vi "Create HTML.vi"(7 "FP Reference":refnum<class "Web Front Panel.lvclass">, 8 "error in (no error)":errorcluster, 10 "VI Identifier":string, 11 "Text In":refnum<class "Text.lvclass">) -> (0 "error out":errorcluster, 1 "js code for controls":string, 2 "js variables":string, 3 "Text Out":refnum<class "Text.lvclass">, 4 "script dependencies":string[](array[string]), 5 "HTML":string, 6 "js code for indicators":string)   [LabVIEW 2017, in "Front Panel Publisher.lvlib" / "Text.lvclass"]
uses:
  Text.lvclass
  Object_class/Object.lvclass
  Front Panel Publisher.lvlib
  String_class/String.lvclass
  Web Front Panel_class/Web Front Panel.lvclass
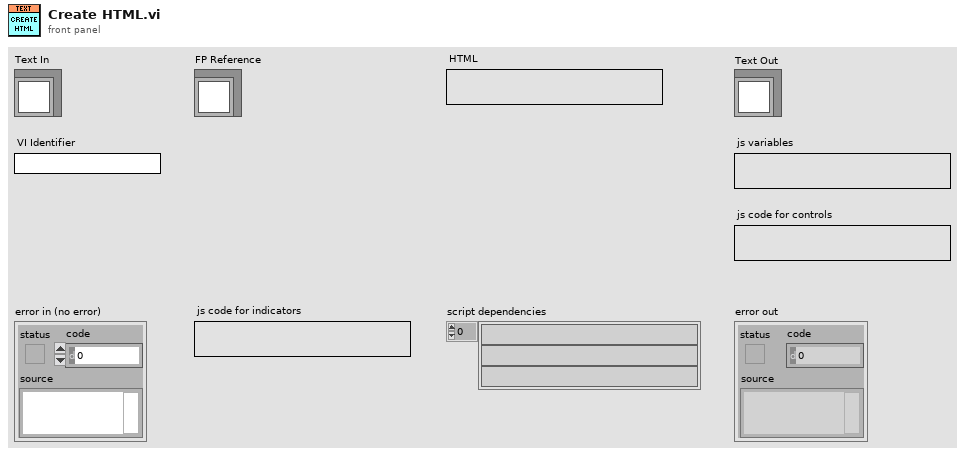
[diagram p1: front panel]
types:
  T1 = typedef "Front Panel Publisher.lvlib/Object.lvclass/Attributes.ctl" = cluster{"UID":i32, "Type":string, "Starting Location":T2, "Reference":refnum<vi>, "Cluster Component":bool, "Starting Rect Position":cluster{"Left":i16, "Top":i16}, "Owning Pane":refnum<vi>, "Master Total Rect Delta":T3}
  T2 = typedef "Front Panel Publisher.lvlib/Object.lvclass/Coordinates.ctl" = cluster{"Left":i32, "Top":i32, "Height":u32, "Width":u32}
  T3 = typedef "LVRectTypeDef.ctl" = cluster{"Left":i16, "Top":i16, "Right":i16, "Bottom":i16}
  T4 = typedef "Front Panel Publisher.lvlib/Text.lvclass/Attributes.ctl" = cluster{"Text":string, "Font":string, "Font Size":u32, "Visible":bool, "Control Reference":refnum<vi>}
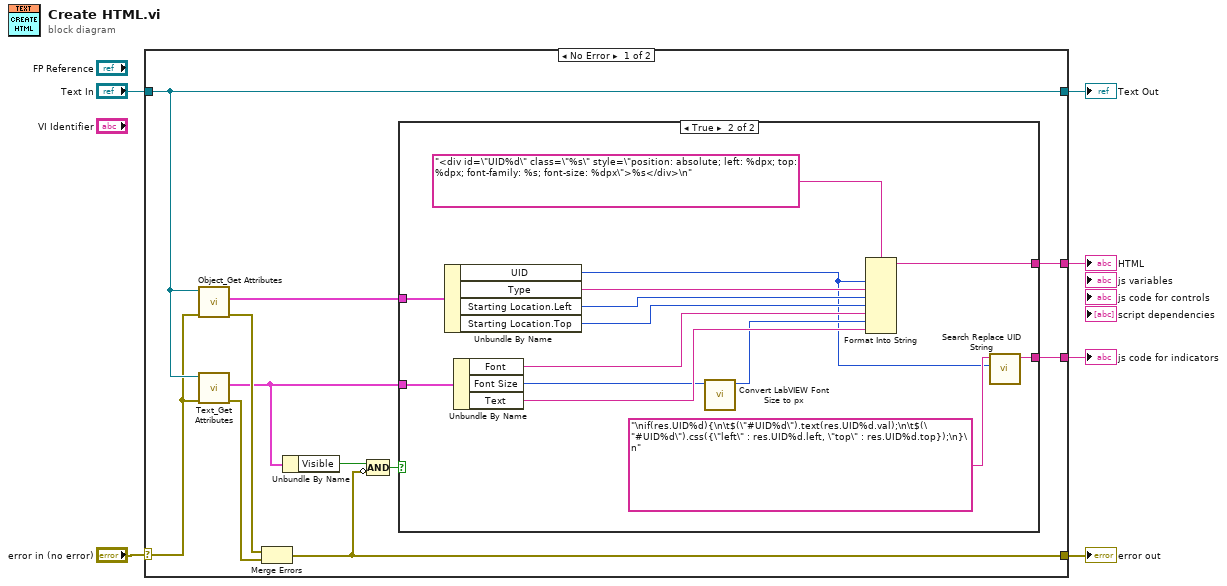
[diagram p0: block diagram]
diagram:
  n1 = case shown="No Error" "error in (no error)" {
    selector: "error in (no error)" -> [w9 w33]
    tunnel: [w15 w33] -> w5
    tunnel: [w13 w32] -> w3
    tunnel: "Text In" -> [w13 w32]
    tunnel: [w14 _] -> w2
    tunnel: [w8 _] -> w1
    frame No Error {
      n2 = call "Object_Get Attributes.vi"("error in (no error)"=w9, "Object In"=w13) -> ("error out"=w16:errorcluster, "Object Attributes"=w7:T1)  [unwired: 7 in, 1 out]
      n3 = call "Text_Get Attributes.vi"("error in (no error)"=w9, "Text In"=w13) -> ("error out"=w17:errorcluster, "Data"=w12:T4)  [unwired: 7 in, 1 out]
      n4 = Merge Errors(w16, w17) -> (w15:errorcluster)
      n5 = Unbundle By Name(w12) -> ("Visible"=w11:bool)
      n6 = Compound Arithmetic op=AND(w11, invert w15) -> (w10:bool)
      n7 = case shown="True" w10 {
        tunnel: [_ w29] -> w14
        tunnel: w12 -> [_ w28]
        tunnel: [_ w23] -> w8
        tunnel: w7 -> [_ w20]
        frame False {
        }
        frame True {
          n8 = Unbundle By Name(w20) -> ("UID"=w18:i32, "Type"=w19:string, "Starting Location.Left"=w31:i32, "Starting Location.Top"=w30:i32)
          n9 = Unbundle By Name(w28) -> ("Font"=w26:string, "Font Size"=w22:u32, "Text"=w27:string)
          n10 = call "Convert LabVIEW Font Size to px.vi"("LabVIEW Font Size"=w22) -> ("px Font Size"=w21:i32)  [unwired: 10 in]
          n11 = Format Into String(format string="<div id=\"UID%d\" class=\"%s\" style=\"position: absolute; left: %dpx; top: %dpx; font-family: %s; font-size: %dpx\">%s</div>\n", w18, w19, w31, w30, w26, w21, w27) -> (resulting string=w29:string)  [unwired: 2 in, 1 out]
          n12 = call "Search Replace UID String.vi"("UID"=w18, "Input String"="\nif(res.UID%d){\n\t$(\"#UID%d\").text(res.UID%d.val);\n\t$(\"#UID%d\").css({\"left\" : res.UID%d.left, \"top\" : res.UID%d.top});\n}\n") -> ("Output String"=w23:string)  [unwired: 9 in]
        }
      }
    }
    frame Error {
    }
  }
  "error out" <- w5
  "Text Out" <- w3
  "HTML" <- w2
  "js code for indicators" <- w1
